vi "LMS_Set_Digital_LPFBW.vi"(4 "enabled":i8, 6 "bandwidth":dbl, 8 "error in (no error)":errorcluster, 9 "chan":u64, 10 "dir_tx":u8, 11 "device_In":i64) -> (0 "error out":errorcluster, 3 "device_Out":i64)   [LabVIEW 2018, in "LMS_LV_Drv.lvlib"]
uses:
  LMS_LV_Drv.lvlib
  C:/Program Files/PothosSDR/bin/LimeSuite.dll
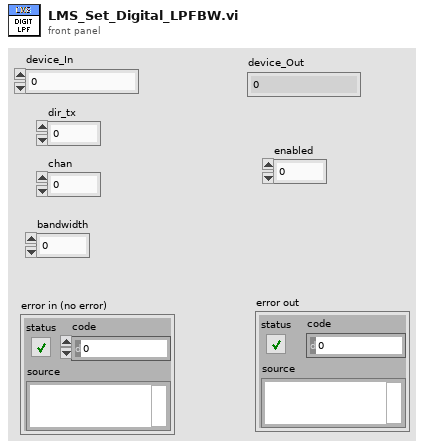
[diagram p1: front panel]
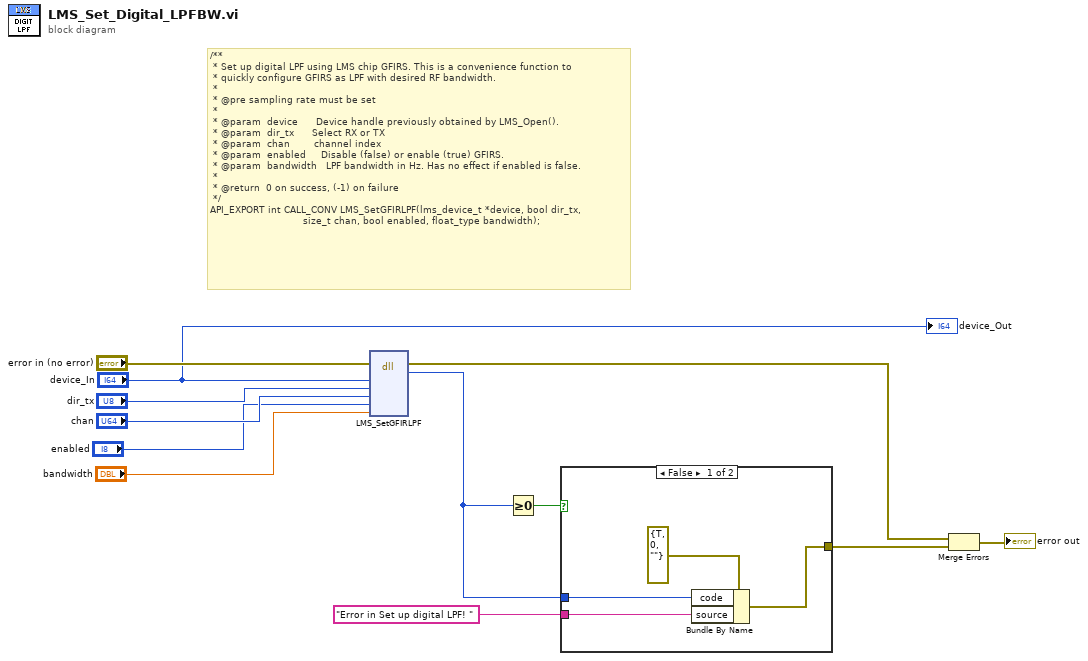
[diagram p0: block diagram]
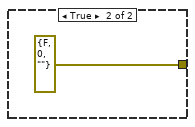
[diagram p2: hidden frame]
diagram:
  # "/**\n * Set up digital LPF using LMS chip GFIRS. This is a convenience function to\n * quickly configure GFIRS as LPF with desired RF bandwidth.\n *\n * @pre sampling rate must be set\n *\n * @param  device      Device handle previously obtained by LMS_Open().\n * @param  dir_tx      Select RX or TX\n * @param  chan        channel index\n * @param  enabled     Disable (false) or enable (true) GFIRS.\n * @param  bandwidth   LPF bandwidth in Hz. Has no effect if enabled is false.\n *\n * @return  0 on success, (-1) on failure\n */\nAPI_EXPORT int CALL_CONV LMS_SetGFIRLPF(lms_device_t *device, bool dir_tx,\n                               size_t chan, bool enabled, float_type bandwidth);"
  n1 = dll-call lib="C:/Program Files/PothosSDR/bin/LimeSuite.dll" fn="LMS_SetGFIRLPF"(error in="error in (no error)", "device"="device_In", "dir_tx"="dir_tx", "chan"="chan", "enabled"="enabled", "bandwidth"="bandwidth") -> (error out=w3:errorcluster, "return type"=w4:i32)  [unwired: 7 in, 1 out]
  n2 = Greater Or Equal To 0?(x=w4) -> (x >= 0?=w7:bool)
  n3 = case shown="False" w7 {
    tunnel: [w15 errorcluster {"status"=FALSE, "code"=0, "source"=""} ("error in")] -> w5
    tunnel: w4 -> [w14 _]
    tunnel: "Error in Set up digital LPF! " ("source") -> [w13 _]
    frame False {
      n4 = Bundle By Name(cluster=errorcluster {"status"=TRUE, "code"=0, "source"=""} ("error in"), "code"=w14, "source"=w13) -> (w15:errorcluster)
    }
    frame True {
    }
  }
  n5 = Merge Errors(w3, w5) -> (→"error out":errorcluster)
  "device_Out" <- "device_In"
